vi "Efecte_Audio.vi"(9 "Activare Ecou":bool, 10 "Activare Tremolo":bool, 11 "Semnal Intrare":dynamicdata(graph) caption="Sine") -> (3 "Semnal Iesire":dynamicdata(graph))   [LabVIEW 2026]
uses:
  <vilib>/Waveform/WDTOps.llb/WDT Append Waveforms DBL.vi
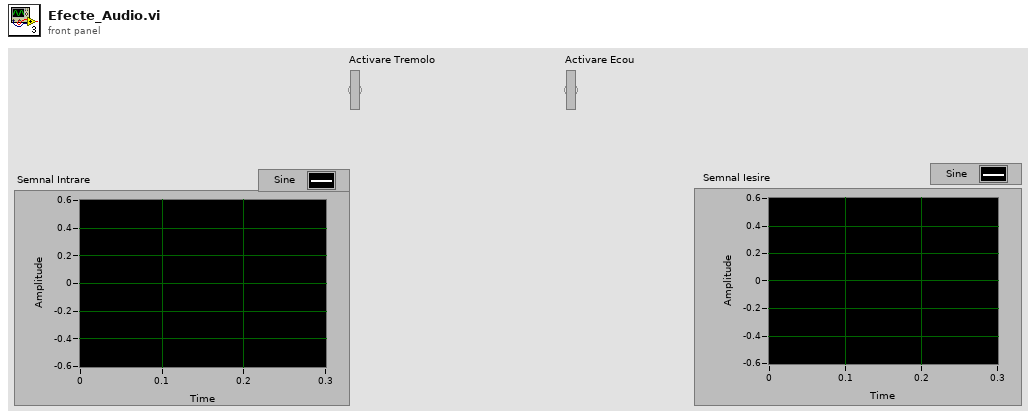
[diagram p1: front panel]
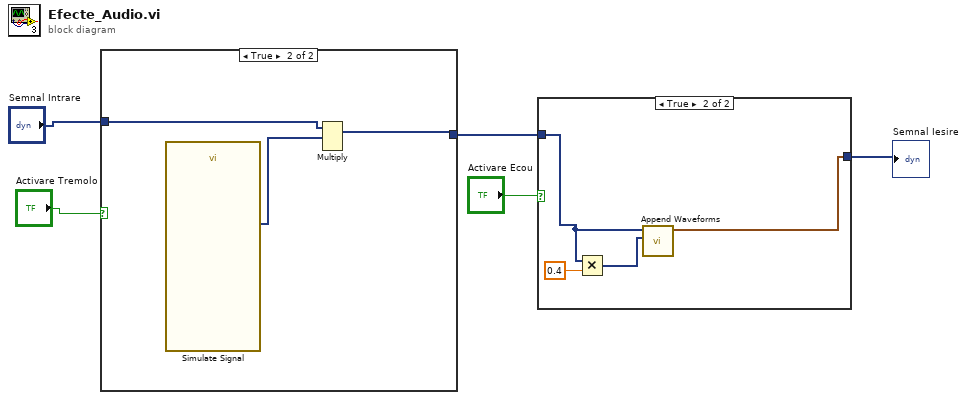
[diagram p0: block diagram]
diagram:
  n1 = case shown="True" "Activare Tremolo" {
    tunnel: [w6 w8] -> w2
    tunnel: "Semnal Intrare" -> [w6 w7]
    frame False {
    }
    frame True {
      n2 = call "Simulate Signal"() -> ("Sine"=w9:dynamicdata)  [unwired: 14 in, 1 out]
      n3 = Multiply(1:w9, 2:w7) -> (0:w8:dynamicdata)  [unwired: 1 in, 1 out]
    }
  }
  n4 = case shown="True" "Activare Ecou" {
    tunnel: w2 -> [w10 w13]
    tunnel: [w10 w11] -> w1
    frame False {
    }
    frame True {
      n5 = Multiply(x=w13, y=0.4) -> (x*y=w12:dynamicdata)
      n6 = call-poly <vilib>:"Append Waveforms.vi"("waveform B"=w12, "waveform A"=w13) -> ("waveform out"=w11:waveform(dbl))  [unwired: 8 in, 1 out]
    }
  }
  "Semnal Iesire" <- w1
